vi "close USB.vi"(8 "error in (no error)":errorcluster caption="错误输入（无错误）") -> (0 "error out":errorcluster caption="错误输出", 3 "function return":i32)   [LabVIEW 2018, in "恒凯采集卡.lvlib"]
doc: "int closeUSB(void);"
uses:
  Usb_Daq_V52_32.dll
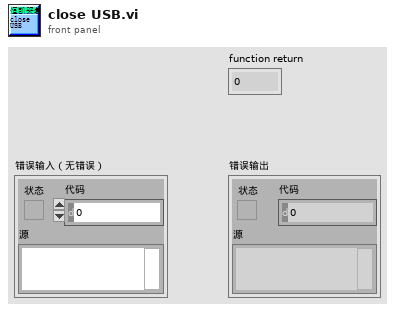
[diagram p1: front panel]
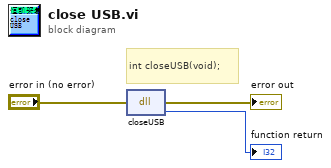
[diagram p0: block diagram]
diagram:
  # "int closeUSB(void);"
  n1 = dll-call lib="PTH2Sabs CUsersLenovoDesktop 心肌细胞电信号_231128 -enUsb_Daq_V52_32.*" fn="closeUSB"(error in="error in (no error)") -> (error out=→"error out":errorcluster, →"function return":i32)  [unwired: 2 in, 1 out]
